vi "Conversão Pressão - kPa.vi"(1 "MIN":i32=-50, 2 "MAX":i32=50, 3 "input":dbl[](array[numeric])) -> (0 "output":dbl[](array[numeric]))   [LabVIEW 2019]
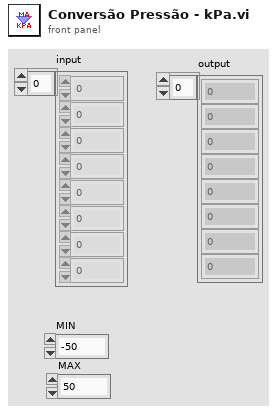
[diagram p1: front panel]
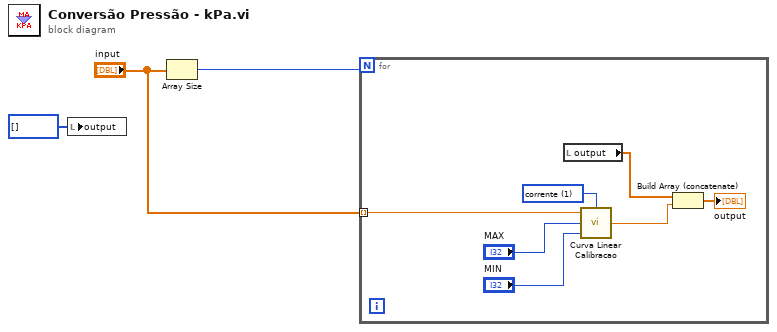
[diagram p0: block diagram]
diagram:
  n1 = local write "output"(i32[] [] ("output")) -> ()
  n2 = Array Size(array="input") -> (size(s)=w3:i32)
  n3 = for {
    N: w3 -> [_]
    tunnel: "input" -> [w6] mode=indexing
    w4 = u16 1 items=["tensao", "corrente"] ("input type")
    n4 = local read "output"() -> (w9:dbl[])
    n5 = call "Curva Linear Calibracao.vi"("input type"=w4, "MIN"="MIN", "MAX"="MAX", "input"=w6) -> ("output"=w5:dbl)
    n6 = Build Array (concatenate)(w9, w5) -> (→"output":dbl[])
  }
